vi "Actor Core.vi"(8 "error in":errorcluster, 11 "Nested in":refnum<class "Generador.lvclass">) -> (0 "error out":errorcluster, 3 "Actor out":refnum<class "Actor.lvclass">)   [LabVIEW 2020, in "Generador señal.lvlib" / "Generador.lvclass"]
doc: "(<B>Filename</B>: Actor Framework.lvlib:Actor.lvclass:Actor Core.vi)\n\nReceives messages to the actor, reacts to them, and initiates any error handling that may shut the actor down.\n\nDescendant classes may override this VI to append parallel tasks for the actor to complete while it handles messages. Overrides use the Call Parent Method node."
uses:
  Generador.lvclass
  C:/Program Files (x86)/National Instruments/LabVIEW 2020/vi.lib/ActorFramework/Actor/Actor.lvclass
  <vilib>/ActorFramework/Actor/Actor.lvclass
  ACQ Generador/ACQ Generador.lvclass
  Generador.lvclass/Generador.ctl
  <vilib>/ActorFramework/Actor/Actor.lvclass/Actor.ctl
  <vilib>/ActorFramework/Message Enqueuer/Message Enqueuer.lvclass/Message Enqueuer.ctl
  Generador Messages/Start Stop ACQ Msg/Start Stop ACQ Msg.lvclass/Start Stop ACQ Msg.ctl
  Generador Messages/Signal Select Msg/Signal Select Msg.lvclass/Signal Select Msg.ctl
  Generador Messages/Write Save Enable Msg/Write Save Enable Msg.lvclass/Write Save Enable Msg.ctl
  Generador Messages/Path gen Msg/Path gen Msg.lvclass/Path gen Msg.ctl
  Generador Messages/File Type Msg/File Type Msg.lvclass/File Type Msg.ctl
  Generador Messages/Amplitude Msg/Amplitude Msg.lvclass/Amplitude Msg.ctl
  Generador Messages/Frequency ACQ Msg/Frequency ACQ Msg.lvclass/Frequency ACQ Msg.ctl
  <vilib>/ActorFramework/Message Enqueuer/Init from Existing Queue.vi
  <vilib>/ActorFramework/Message Enqueuer/Enqueue.vi
  <vilib>/ActorFramework/Stop Msg/Stop Msg.lvclass
  C:/Program Files (x86)/National Instruments/LabVIEW 2020/vi.lib/ActorFramework/Message/Message.lvclass
  Generador Messages/Start Stop ACQ Msg/Start Stop ACQ Msg.lvclass
  Generador Messages/Signal Select Msg/Signal Select Msg.lvclass
  Generador Messages/Write Save Enable Msg/Write Save Enable Msg.lvclass
  Generador Messages/Path gen Msg/Path gen Msg.lvclass
  Generador Messages/File Type Msg/File Type Msg.lvclass
  Generador Messages/Amplitude Msg/Amplitude Msg.lvclass
  Generador Messages/Frequency ACQ Msg/Frequency ACQ Msg.lvclass
  <vilib>/ActorFramework/Message Priority Queue/Priority Enqueue.vi
  <vilib>/ActorFramework/Message Enqueuer/Message Enqueuer.lvclass
panel:
  out "Waveform Graph":waveform(dbl)(graph)
  in  "Frequency":dbl
  in  "Amplitude":dbl
  in  "Signal":u16(ring) items=["Senoidal", "Cuadrada", "Triangular"]
  in  "File Type":u16(ring) items=["Text", "CSV"]
  in  "File Path":path
  in  "Save Button":bool
  in  "Stop":bool
  in  "Start":bool
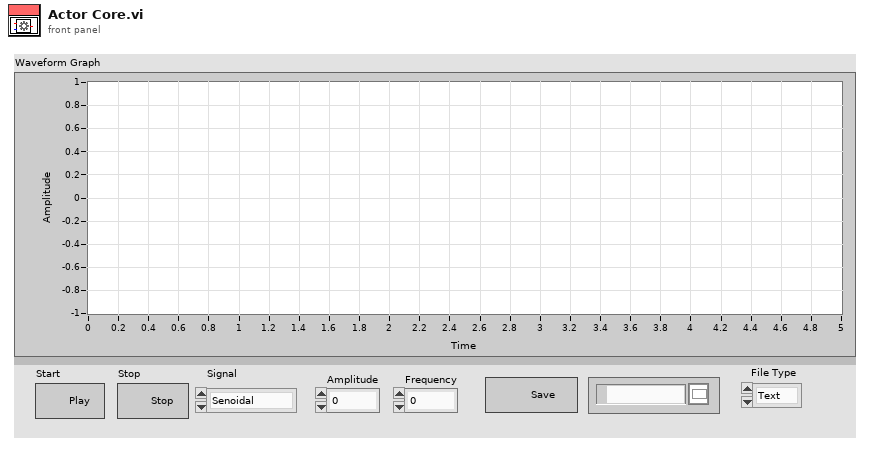
[diagram p1: front panel]
types:
  T1 = enum8{"Enabled", "Disabled", "Disabled and Grayed Out"}
  T2 = cluster{"Stop":refnum<user-event>, "Waveform Chart":refnum<user-event>}
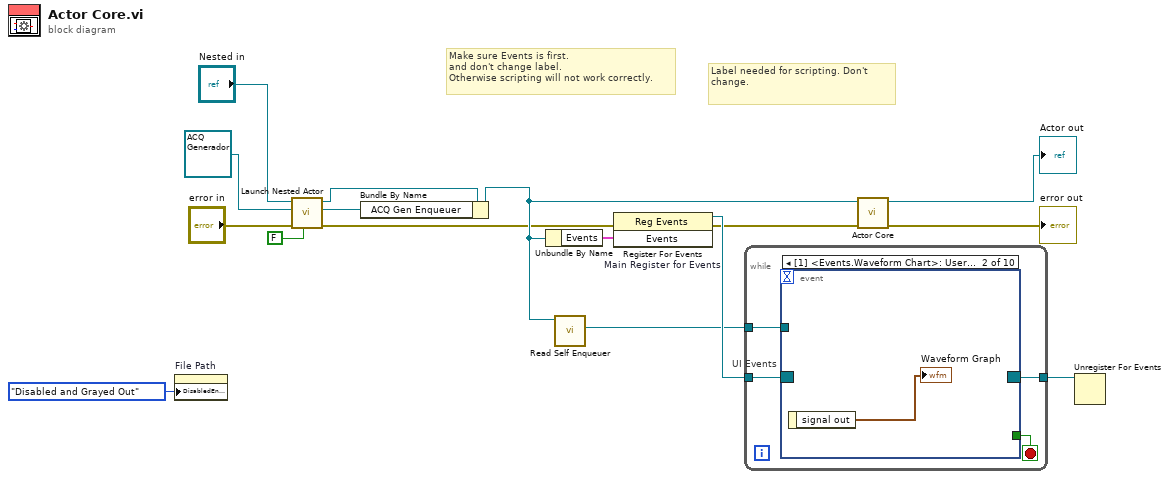
[diagram p0: block diagram]
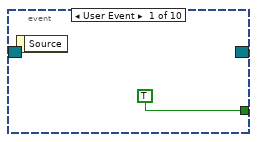
[diagram p2: hidden frame]
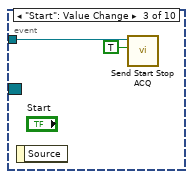
[diagram p3: hidden frame]
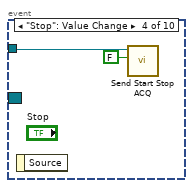
[diagram p4: hidden frame]
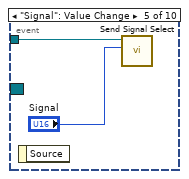
[diagram p5: hidden frame]
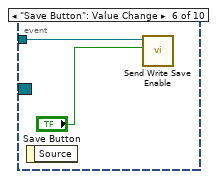
[diagram p6: hidden frame]
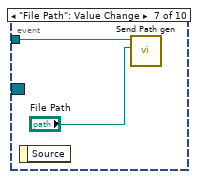
[diagram p7: hidden frame]
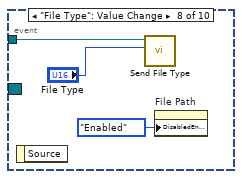
[diagram p8: hidden frame]
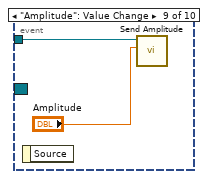
[diagram p9: hidden frame]
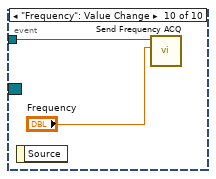
[diagram p10: hidden frame]
diagram:
  # "Label needed for scripting. Don't change."
  # "Make sure Events is first.\nand don't change label.\nOtherwise scripting will not work correctly."
  n1 = property on="File Path" class="Path"("DisabledEnum"=T1."Disabled and Grayed Out" ("Disabled")) -> ()  [unwired: 2 in, 2 out]
  n2 = call <vilib>:"Launch Nested Actor.vi"("Open Actor Core front panel? (F)"=FALSE, "error in (no error)"="error in", "Nested Actor"=refnum<class "ACQ Generador.lvclass"> refnum ("ACQ Generador.lvlib:ACQ Generador.lvclass"), "Caller Actor in"="Nested in") -> ("error out"=w2:errorcluster, "Nested Actor's Enqueuer"=w5:refnum<class "Message Enqueuer.lvclass">, "Caller Actor out"=w7:refnum<class "Generador.lvclass">)  [unwired: 5 in]
  n3 = Bundle By Name(cluster=w7, "ACQ Gen Enqueuer"=w5) -> (w6:refnum<class "Generador.lvclass">)
  n4 = Unbundle By Name(w6) -> ("Events"=w13:T2)
  n5 = call <vilib>:"Read Self Enqueuer.vi"("Actor"=w6) -> ("Self Enqueuer"=w11:refnum<class "Message Enqueuer.lvclass">)  [unwired: 10 in]
  n6 = register-events "Main Register for Events"(error in=w2, w13) -> (reference out=w14:refnum<event-registration>, error out=w10:errorcluster)  [unwired: 1 in]
  n7 = while {
    tunnel: w14 -> [w20]
    tunnel: [w18] -> w12
    tunnel: w11 -> [w17]
    stop <- w19 stop-if-true
    n8 = event "UI Events" shown="[1] <Events.Waveform Chart>: User Event" {
      selector: w20 -> [_ _ _ _ _ _ _ _ _ _]
      dyn-events: [_ _ _ _ _ _ _ _ _ _] -> w18
      timeout: _ -> [_ _ _ _ _ _ _ _ _ _]
      tunnel: [TRUE _ _ _ _ _ _ _ _ _] -> w19
      tunnel: w17 -> [_ _ w24 w26 w28 w30 w32 w34 w37 w39]
      event User Event {
        n9 = event-data() -> ()  [unwired: 1 in, 1 out]
      }
      event User Event {
        n10 = event-data() -> ("signal out"=→"Waveform Graph":waveform(dbl))  [unwired: 1 in]
      }
      event "Start": Value Change {
        n11 = event-data() -> ()  [unwired: 1 in, 1 out]
        n12 = call "Send Start Stop ACQ.vi"("Start/Stop"=TRUE, "Message Enqueuer"=w24) -> ()  [unwired: 8 in, 2 out]
      }
      event "Stop": Value Change {
        n13 = event-data() -> ()  [unwired: 1 in, 1 out]
        n14 = call "Send Start Stop ACQ.vi"("Start/Stop"=FALSE, "Message Enqueuer"=w26) -> ()  [unwired: 8 in, 2 out]
      }
      event "Signal": Value Change {
        n15 = event-data() -> ()  [unwired: 1 in, 1 out]
        n16 = call "Send Signal Select.vi"("Signal"="Signal", "Message Enqueuer"=w28) -> ()  [unwired: 8 in, 2 out]
      }
      event "Save Button": Value Change {
        n17 = event-data() -> ()  [unwired: 1 in, 1 out]
        n18 = call "Send Write Save Enable.vi"("Save Enable"="Save Button", "Message Enqueuer"=w30) -> ()  [unwired: 8 in, 2 out]
      }
      event "File Path": Value Change {
        n19 = event-data() -> ()  [unwired: 1 in, 1 out]
        n20 = call "Send Path gen.vi"("Path"="File Path", "Message Enqueuer"=w32) -> ()  [unwired: 8 in, 2 out]
      }
      event "File Type": Value Change {
        n21 = event-data() -> ()  [unwired: 1 in, 1 out]
        n22 = call "Send File Type.vi"("File Type"="File Type", "Message Enqueuer"=w34) -> ()  [unwired: 8 in, 2 out]
        n23 = property on="File Path" class="Path"("DisabledEnum"=T1."Enabled" ("Disabled")) -> ()  [unwired: 2 in, 2 out]
      }
      event "Amplitude": Value Change {
        n24 = event-data() -> ()  [unwired: 1 in, 1 out]
        n25 = call "Send Amplitude.vi"("Amplitude"="Amplitude", "Message Enqueuer"=w37) -> ()  [unwired: 8 in, 2 out]
      }
      event "Frequency": Value Change {
        n26 = event-data() -> ()  [unwired: 1 in, 1 out]
        n27 = call "Send Frequency ACQ.vi"("Frequency"="Frequency", "Message Enqueuer"=w39) -> ()  [unwired: 8 in, 2 out]
      }
    }
  }
  n28 = call-parent "Actor Core.vi"("error in"=w10, "Actor in"=w6) -> ("error out"=→"error out":errorcluster, "Actor out"=→"Actor out":refnum<class "Actor.lvclass">)  [unwired: 8 in]
  n29 = Unregister For Events(event registration refnum=w12) -> ()  [unwired: 1 in, 1 out]
